vi "digital integration.vi"() -> ()   [LabVIEW 2017]
uses:
  <vilib>/measure/NI_MABase.lvlib
panel:
  in  "signal type 3":T1(ring)
  in  "frequency 3":dbl=10.0 format="%0.2p"
  in  "signal type 4":T1(ring)
  in  "frequency 4":dbl=10.0 format="%0.2p"
  out "mq6 voltage":dbl
  out "flame voltage":dbl
  out "Waveform Chart":dynamicdata(graph)
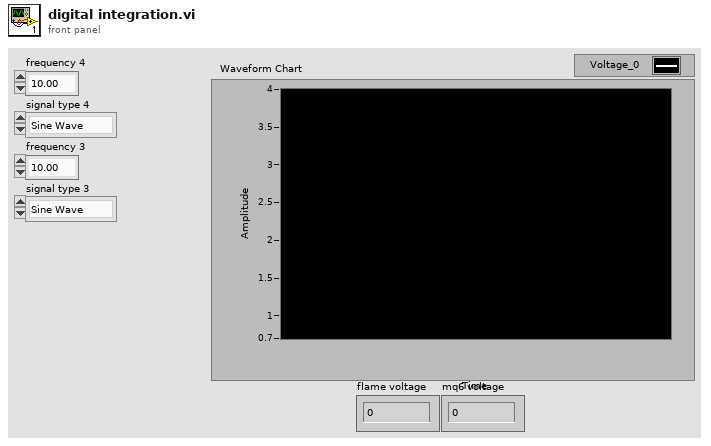
[diagram p1: front panel]
types:
  T1 = enum16{"Sine Wave", "Triangle Wave", "Square Wave", "Sawtooth Wave"}
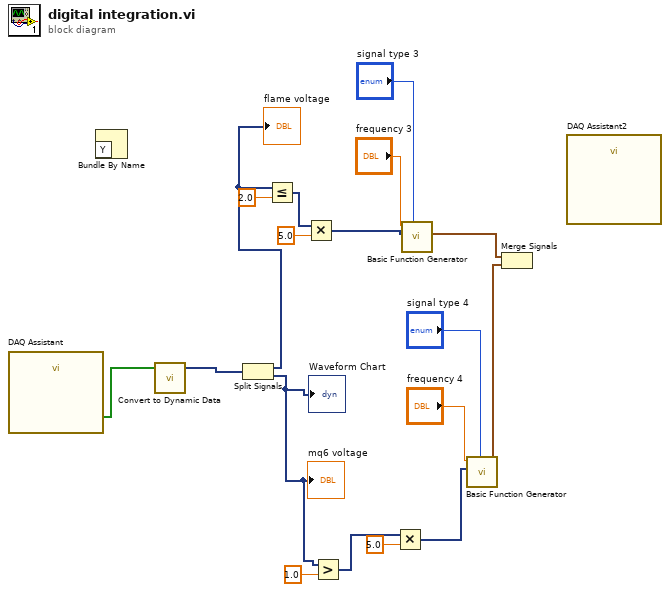
[diagram p0: block diagram]
diagram:
  n1 = call "DAQ Assistant"() -> ("data"=w2:bool[])  [unwired: 17 in, 2 out]
  n2 = Bundle By Name() -> ()  [unwired: 2 in, 1 out]
  n3 = call "Convert to Dynamic Data"("Array"=w2) -> ("Dynamic Data Type"=w1:dynamicdata)  [unwired: 3 in]
  n4 = Split Signals(w1) -> (w8:dynamicdata, w14:dynamicdata)  [unwired: 2 in]
  "Waveform Chart" <- w14
  "flame voltage" <- w8
  "mq6 voltage" <- w14
  n5 = Less Or Equal?(x=w8, y=2.0) -> (x <= y?=w7:dynamicdata)
  n6 = Multiply(x=w7, y=5.0) -> (x*y=w6:dynamicdata)
  n7 = Greater?(x=w14, y=1.0) -> (0:w13:dynamicdata)
  n8 = Multiply(x=w13, y=5.0) -> (x*y=w12:dynamicdata)
  n9 = call <vilib>:"Basic Function Generator.vi"("signal type"="signal type 3", "amplitude"=w6, "frequency"="frequency 3") -> ("signal out"=w3:waveform(dbl))  [unwired: 6 in, 2 out]
  n10 = call <vilib>:"Basic Function Generator.vi"("signal type"="signal type 4", "amplitude"=w12, "frequency"="frequency 4") -> ("signal out"=w9:waveform(dbl))  [unwired: 6 in, 2 out]
  n11 = Merge Signals(w3, w9) -> ()  [unwired: 1 out]
  n12 = call "DAQ Assistant2"() -> ()  [unwired: 18 in, 2 out]
